vi "Vertical Spacing.vi"() -> (3 "Spacing":i32=42)   [LabVIEW 2020, in "FlexBlocks.lvlib"]
uses:
  FlexBlocks.lvlib
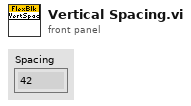
[diagram p1: front panel]
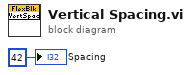
[diagram p0: block diagram]
diagram:
  "Spacing" <- 42
